vi "Read validCmdIsTrue.vi"(11 "CommandConstruction in":refnum<class "CommandConstruction.lvclass">) -> (2 "validCmdIsTrue":bool, 3 "CommandConstruction out":refnum<class "CommandConstruction.lvclass">)   [LabVIEW 2016, in "CommandConstruction.lvclass"]
uses:
  CommandConstruction.lvclass
  CommandConstruction.lvclass/CommandConstruction.ctl
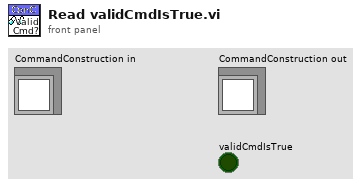
[diagram p1: front panel]
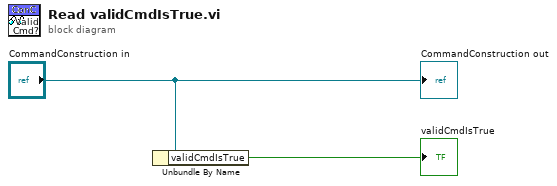
[diagram p0: block diagram]
diagram:
  n1 = Unbundle By Name("CommandConstruction in") -> ("validCmdIsTrue"=→"validCmdIsTrue":bool)
  "CommandConstruction out" <- "CommandConstruction in"
